vi "Handle Command.vi"(8 "error in":errorcluster, 10 "CMD In":refnum<class "Change Speaker Vparams.lvclass">, 11 "Object In":refnum<class>) -> (0 "error out":errorcluster, 1 "Command Successful?":bool, 2 "CMD Out":refnum<class "Change Speaker Vparams.lvclass">, 3 "Object Out":refnum<class>)   [LabVIEW 2018, in "ePAS Library.lvlib" / "Change Speaker Vparams.lvclass"]
doc: "Abstract method for accomplishing the execution of a command directed to an instrument object on the wire."
uses:
  Change Speaker Vparams.lvclass
  Instrument/ePAS.lvclass
  C:/Users/Labview/Documents/exscalabar_server/reusable/Instrument/Instrument.lvclass
  Instrument/ePAS.lvclass/ePAS.ctl
  reusable/Instrument/Instrument.lvclass/Instrument.ctl
  Change Speaker Vparams.lvclass/Change Speaker Vparams.ctl
  Instrument/Accessors/Read FPGA Session.vi
  reusable/Instrument/Read Log Session.vi
  reusable/Instrument/Read ExtCom.vi
  <vilib>/Utility/error.llb/Error Cluster From Error Code.vi
  <vilib>/rvi/errors/niLvFpgaAdjustHostInterfaceError.vi
  <userlib>/_Session Fwk/Session - Root.lvclass
  <vilib>/rvi/interface/nirviReadWriteControl/nirviReadWriteControl.xnode
  FPGA/R FPGA Ref.ctl
  FPGA Bitfiles/FPGAServer.lvbitx
  FPGA/Session/Exscalabar FPGA.lvclass
  ePAS Library.lvlib
  reusable/Session APIs/Session Log/System Log.lvclass
  NiFpgaLv.dll
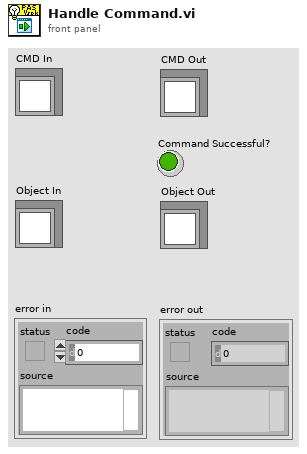
[diagram p1: front panel]
types:
  T1 = typedef "Session - Root.lvclass/Session Handle.ctl" = refnum<data-value>
  T2 = typedef "ePAS Library.lvlib/R FPGA Ref.ctl" = refnum<k20>
  T3 = cluster{"tag":string, "section":string, "data":variant}
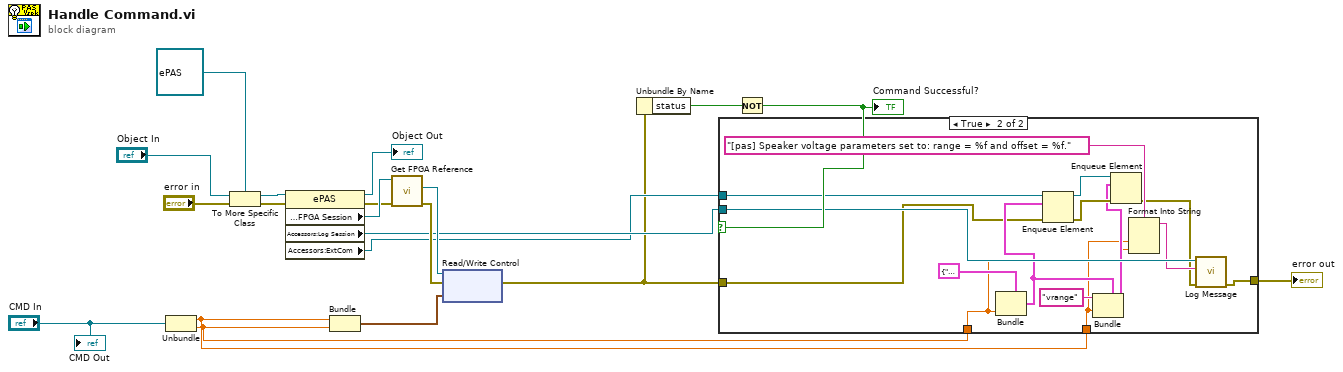
[diagram p0: block diagram]
diagram:
  n1 = Unbundle("CMD In") -> (w3:dbl, w4:dbl)
  n2 = To More Specific Class(target class=refnum<class "ePAS.lvclass"> refnum ("ePAS"), reference="Object In", error in="error in") -> (specific class reference=w19:refnum<class "ePAS.lvclass">, error out=w20:errorcluster)
  n3 = property class="ePAS"(reference=w19, error in=w20) -> (reference out=→"Object Out":refnum<class "ePAS.lvclass">, error out=w16:errorcluster, "Accessors:FPGA Session"=w17:T1, "Accessors:Log Session"=w6:T1, "Accessors:ExtCom"=w5:refnum<queue>)
  n4 = Bundle("Vrange"=w3, "Voffset"=w4) -> (w9:cluster{"Vrange":dbl, "Voffset":dbl})  [unwired: 1 in]
  n5 = call "Get FPGA Reference.vi"("error in"=w16, "Session In"=w17) -> ("error out"=w13:errorcluster, "Ex FPGA Ref"=w14:T2)  [unwired: 7 in, 1 out]
  n6 = xnode "Read/Write Control"("FPGA VI Reference In"=w14, "error in"=w13, "Speaker"=w9) -> ("error out"=w2:errorcluster)  [unwired: 1 out]
  n7 = Unbundle By Name(w2) -> ("status"=w8:bool)
  n8 = Not(x=w8) -> (.not. x?=w7:bool)
  "Command Successful?" <- w7
  n9 = case shown="True" w7 {
    tunnel: w5 -> [_ w36]
    tunnel: w4 -> [_ w24]
    tunnel: w6 -> [_ w34]
    tunnel: w3 -> [_ w25]
    tunnel: w2 -> [w21 w23]
    tunnel: [w21 w22] -> w1
    frame False {
    }
    frame True {
      n10 = Bundle(cluster=T3 {"tag"="voffset", "section"="pas.spk", "data"=variant} ("element"), "data"=w24) -> (w28:T3)  [unwired: 2 in]
      n11 = Enqueue Element(queue=w36, element=w28, error in (no error)=w23) -> (queue out=w29:refnum<queue>, error out=w31:errorcluster)  [unwired: 1 in, 1 out]
      n12 = Bundle(cluster=w28, "tag"="vrange", "data"=w25) -> (w26:T3)  [unwired: 1 in]
      n13 = Enqueue Element(queue=w29, element=w26, error in (no error)=w31) -> (error out=w30:errorcluster)  [unwired: 1 in, 2 out]
      n14 = Format Into String(format string="[pas] Speaker voltage parameters set to: range = %f and offset = %f.", w25, w24) -> (resulting string=w32:string)  [unwired: 2 in, 1 out]
      n15 = call "Log Message.vi"("error in"=w30, "MSG In"=w32, "session in"=w34) -> ("error out"=w22:errorcluster)  [unwired: 7 in, 1 out]
    }
  }
  "error out" <- w1
  "CMD Out" <- "CMD In"
